vi "_match_first_string.vi"(3 "String to match":string, 5 "Array in":string[](array[string])) -> (1 "Index out":i32)   [LabVIEW 2022 SP3, in "hmp4000_rsidr_core.lvlib"]
uses:
  hmp4000_rsidr_core.lvlib
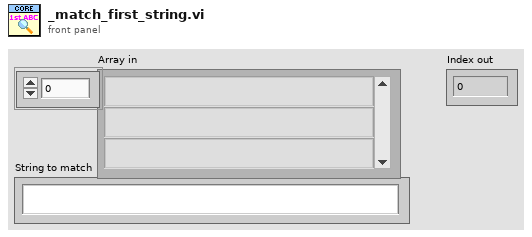
[diagram p1: front panel]
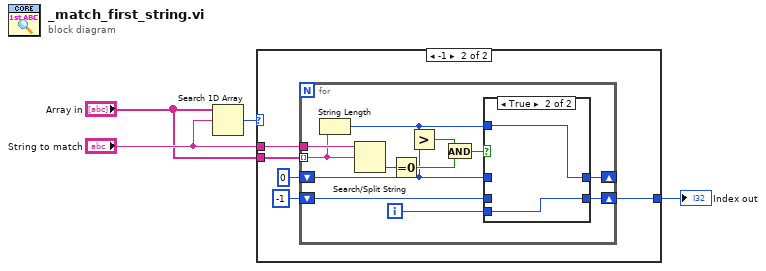
[diagram p0: block diagram]
diagram:
  n1 = Search 1D Array(1D array="Array in", element="String to match") -> (index of element=w3:i32)  [unwired: 1 in]
  n2 = case shown="-1" w3 {
    selector: w3 -> [w5 _]
    tunnel: [w5 w8] -> w4
    tunnel: "Array in" -> [_ w6]
    tunnel: "String to match" -> [_ w7]
    frame 0, Default {
    }
    frame -1 {
      n3 = for {
        tunnel: w6 -> [w20] mode=indexing
        tunnel: w7 -> [w22]
        shift-right: [w12] -> w8
        shift-left: -1 -> [w13]
        shift-right: [w14] -> _
        shift-left: 0 -> [w15]
        i -> [w11]
        n4 = String Length(string=w20) -> (length=w19:i32)
        n5 = Search/Split String(string=w22, search string/char (-)=w20) -> (offset of match=w21:i32)  [unwired: 1 in, 2 out]
        n6 = Equal To 0?(x=w21) -> (x = 0?=w17:bool)
        n7 = Greater?(x=w19, y=w15) -> (0:w18:bool)
        n8 = And(x=w18, y=w17) -> (x .and. y?=w16:bool)
        n9 = case shown="True" w16 {
          tunnel: w19 -> [_ w26]
          tunnel: w15 -> [w24 _]
          tunnel: [w24 w26] -> w14
          tunnel: w13 -> [w23 _]
          tunnel: [w23 w25] -> w12
          tunnel: w11 -> [_ w25]
          frame False {
          }
          frame True {
          }
        }
      }
    }
  }
  "Index out" <- w4
